vi "Untitled 1.vi"() -> ()   [LabVIEW 2010]
uses:
  Control 12.ctl
panel:
  out "х2":dbl
  out "x1":dbl
  out "x":dbl
  out "D":dbl
  in  "Розрахувати":bool
  in  "Вихід":bool
  in  "c":dbl
  in  "b":dbl
  in  "a":dbl
  # "Вхідні дані:"
  # "Результати:"
  # "При D=0 маємо"
  # "При D>0 маємо"
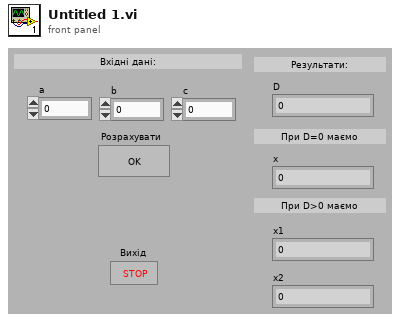
[diagram p1: front panel]
types:
  T1 = cluster{"a":dbl, "b":dbl, "c":dbl, "D":dbl, "x":dbl, "x1":dbl, "x2":dbl}
  T2 = typedef "Control 12.ctl" = enum16{"Розрахувати", "stop", "c", "b", "a"}
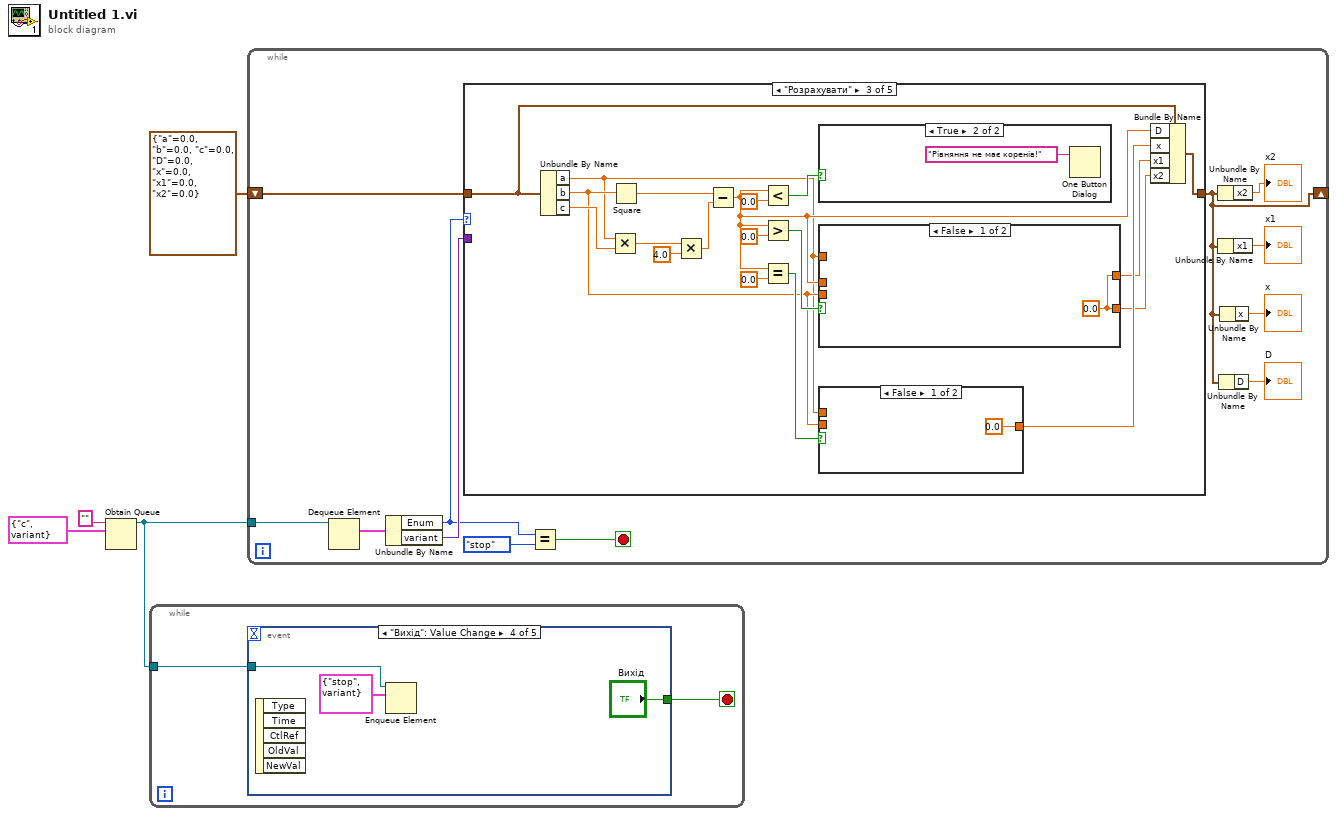
[diagram p0: block diagram]
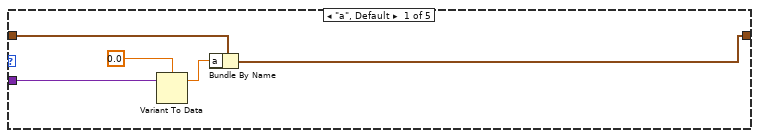
[diagram p2: hidden frame]
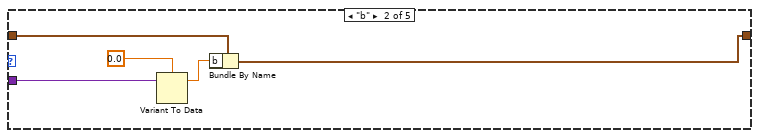
[diagram p3: hidden frame]
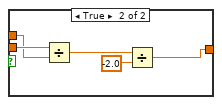
[diagram p5: hidden frame]
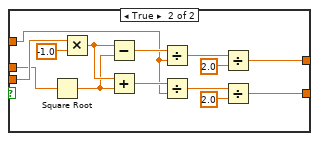
[diagram p6: hidden frame]
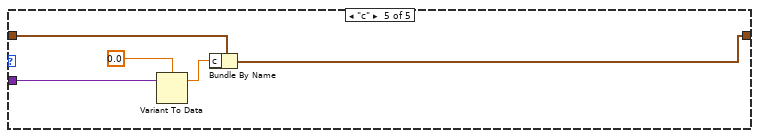
[diagram p8: hidden frame]
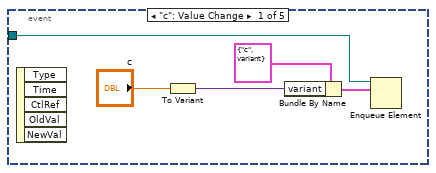
[diagram p9: hidden frame]
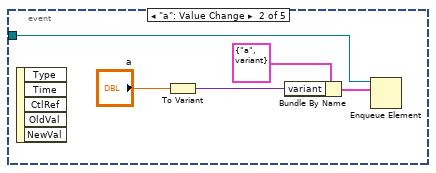
[diagram p10: hidden frame]
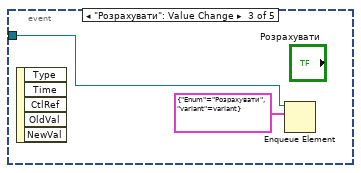
[diagram p11: hidden frame]
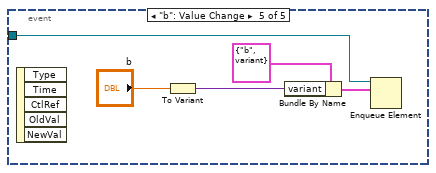
[diagram p12: hidden frame]
diagram:
  n1 = Obtain Queue(name (unnamed)="", element data type=cluster{"Enum":T2, "variant":variant} {"Enum"=enum."c", "variant"=variant}) -> (queue out=w2:refnum<queue>)  [unwired: 3 in, 2 out]
  n2 = while {
    tunnel: w2 -> [w6]
    stop <- w5 stop-if-true
    n3 = event shown="[3] \"Вихід\": Value Change" {
      selector: _ -> [_ _ _ _ _]
      dyn-events: _ -> [_ _ _ _ _]
      timeout: _ -> [_ _ _ _ _]
      tunnel: w6 -> [w11 w16 w18 w19 w26]
      tunnel: [_ _ _ "Вихід" _] -> w5
      event "c": Value Change {
        n4 = event-data() -> ()  [unwired: 1 in, 5 out]
        n5 = To Variant(anything="c") -> (Variant=w10:variant)
        n6 = Bundle By Name(cluster=cluster{"Enum":T2, "variant":variant} {"Enum"=enum."c", "variant"=variant} ("element"), "variant"=w10) -> (w7:cluster{"Enum":T2, "variant":variant})
        n7 = Enqueue Element(queue=w11, element=w7) -> ()  [unwired: 2 in, 3 out]
      }
      event "a": Value Change {
        n8 = event-data() -> ()  [unwired: 1 in, 5 out]
        n9 = To Variant(anything="a") -> (Variant=w14:variant)
        n10 = Bundle By Name(cluster=cluster{"Enum":T2, "variant":variant} {"Enum"=enum."a", "variant"=variant} ("element"), "variant"=w14) -> (w12:cluster{"Enum":T2, "variant":variant})
        n11 = Enqueue Element(queue=w16, element=w12) -> ()  [unwired: 2 in, 3 out]
      }
      event "Розрахувати": Value Change {
        n12 = event-data() -> ()  [unwired: 1 in, 5 out]
        n13 = Enqueue Element(queue=w18, element=cluster{"Enum":T2, "variant":variant} {"Enum"=enum."Розрахувати", "variant"=variant}) -> ()  [unwired: 2 in, 3 out]
      }
      event "Вихід": Value Change {
        n14 = event-data() -> ()  [unwired: 1 in, 5 out]
        n15 = Enqueue Element(queue=w19, element=cluster{"Enum":T2, "variant":variant} {"Enum"=enum."stop", "variant"=variant}) -> ()  [unwired: 2 in, 3 out]
      }
      event "b": Value Change {
        n16 = event-data() -> ()  [unwired: 1 in, 5 out]
        n17 = To Variant(anything="b") -> (Variant=w25:variant)
        n18 = Bundle By Name(cluster=cluster{"Enum":T2, "variant":variant} {"Enum"=enum."b", "variant"=variant} ("element"), "variant"=w25) -> (w22:cluster{"Enum":T2, "variant":variant})
        n19 = Enqueue Element(queue=w26, element=w22) -> ()  [unwired: 2 in, 3 out]
      }
    }
  }
  n20 = while {
    tunnel: w2 -> [w38]
    shift-right: [w29] -> _
    shift-left: T1 {"a"=0.0, "b"=0.0, "c"=0.0, "D"=0.0, "x"=0.0, "x1"=0.0, "x2"=0.0} -> [w32]
    stop <- w34 stop-if-true
    n21 = Dequeue Element(queue=w38) -> (element=w37:cluster{"Enum":T2, "variant":variant})  [unwired: 2 in, 3 out]
    n22 = Unbundle By Name(w37) -> ("Enum"=w35:T2, "variant"=w36:variant)
    n23 = case shown="\"Розрахувати\"" w35 {
      tunnel: w36 -> [w41 w45 _ _ w92]
      tunnel: w32 -> [w43 w48 w52 w90 w95]
      tunnel: [w42 w47 w56 w90 w94] -> w29
      frame "a", Default {
        n24 = Variant To Data(Variant=w41, type=0.0) -> (data=w39:dbl)  [unwired: 1 in, 1 out]
        n25 = Bundle By Name(cluster=w43, "a"=w39) -> (w42:T1)
      }
      frame "b" {
        n26 = Variant To Data(Variant=w45, type=0.0) -> (data=w44:dbl)  [unwired: 1 in, 1 out]
        n27 = Bundle By Name(cluster=w48, "b"=w44) -> (w47:T1)
      }
      frame "Розрахувати" {
        n28 = Unbundle By Name(w52) -> ("a"=w53:dbl, "b"=w55:dbl, "c"=w61:dbl)
        n29 = Multiply(x=w53, y=w61) -> (x*y=w60:dbl)
        n30 = Square(x=w55) -> (x^2=w58:dbl)
        n31 = Multiply(x=w60, y=4.0) -> (x*y=w57:dbl)
        n32 = Subtract(x=w58, y=w57) -> (x-y=w54:dbl)
        n33 = Less?(x=w54, y=0.0) -> (x < y?=w65:bool)
        n34 = Greater?(x=w54, y=0.0) -> (0:w67:bool)
        n35 = Equal?(x=w54, y=0.0) -> (x = y?=w66:bool)
        n36 = case shown="True" w65 {
          frame False {
          }
          frame True {
            n37 = One Button Dialog(message="Рівняння не має коренів!") -> ()  [unwired: 1 in, 1 out]
          }
        }
        n38 = case shown="False" w67 {
          tunnel: w55 -> [_ w89]
          tunnel: w54 -> [_ w87]
          tunnel: w53 -> [_ w81]
          tunnel: [w75 w77] -> w50
          tunnel: [w75 w76] -> w49
          frame False {
            w75 = 0.0 ("y")
          }
          frame True {
            n39 = Square Root(x=w87) -> (sqrt(x)=w83:dbl)
            n40 = Multiply(x=w89, y=-1.0) -> (x*y=w84:dbl)
            n41 = Subtract(x=w84, y=w83) -> (x-y=w86:dbl)
            n42 = Add(x=w84, y=w83) -> (x+y=w82:dbl)
            n43 = Divide(x=w86, y=w81) -> (x/y=w85:dbl)
            n44 = Divide(x=w82, y=w81) -> (x/y=w79:dbl)
            n45 = Divide(x=w85, y=2.0) -> (x/y=w77:dbl)
            n46 = Divide(x=w79, y=2.0) -> (x/y=w76:dbl)
          }
        }
        n47 = case shown="False" w66 {
          tunnel: w55 -> [_ w74]
          tunnel: w53 -> [_ w73]
          tunnel: [0.0 ("y") w70] -> w51
          frame False {
          }
          frame True {
            n48 = Divide(x=w74, y=w73) -> (x/y=w72:dbl)
            n49 = Divide(x=w72, y=-2.0) -> (x/y=w70:dbl)
          }
        }
        n50 = Bundle By Name(cluster=w52, "D"=w54, "x"=w51, "x1"=w50, "x2"=w49) -> (w56:T1)
      }
      frame "stop" {
      }
      frame "c" {
        n51 = Variant To Data(Variant=w92, type=0.0) -> (data=w91:dbl)  [unwired: 1 in, 1 out]
        n52 = Bundle By Name(cluster=w95, "c"=w91) -> (w94:T1)
      }
    }
    n53 = Equal?(x=w35, y=Control_12."stop" ("Enum")) -> (x = y?=w34:bool)
    n54 = Unbundle By Name(w29) -> ("x2"=→"х2":dbl)
    n55 = Unbundle By Name(w29) -> ("x1"=→"x1":dbl)
    n56 = Unbundle By Name(w29) -> ("D"=→"D":dbl)
    n57 = Unbundle By Name(w29) -> ("x"=→"x":dbl)
  }
